vi "Add Peak and Valley Detection Settings Section.vi"(8 "error in (no error)":errorcluster, 10 "Stages":string[](array[string])=["Boost", "Battery", "Off"], 11 "Global Settings Item Ref in":T1=18446744073709551615 format="%.0x") -> (0 "error out":errorcluster, 3 "Global Settings Item Ref out":T1=18446744073709551615 format="%.0x")   [LabVIEW 2015, in "Fuel Injector Analysis Addon System Explorer.lvlib"]
uses:
  Fuel Injector Analysis Addon System Explorer.lvlib
  <vilib>/NI Veristand/Custom Device API/Custom Device Item Ref.ctl
  Shared/Types/Analysis.Channels.Select.ctl
  <vilib>/NI Veristand/Custom Device API/Custom Device Channel.ctl
  <vilib>/NI Veristand/Custom Device API/Custom Device Channel Type.ctl
  Shared/Types/Stage.PullIn.Types.ctl
  Shared/Types/Stage.Transition.Types.ctl
  Shared/Constants.vi
  <vilib>/NI Veristand/Custom Device Tools/Custom Device Utility Library/NI VeriStand - Search for Item by GUID.vi
  <vilib>/NI Veristand/Custom Device API/Custom Device API.lvlib
  Shared/Fuel Injector Analysis Addon Shared.lvlib
  <vilib>/NI Veristand/Custom Device Tools/Custom Device Utility Library/Custom Device Utility Library.lvlib
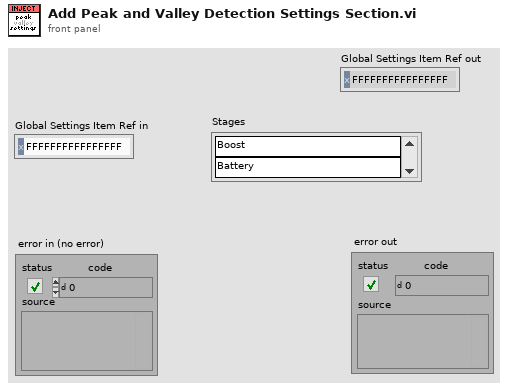
[diagram p1: front panel]
types:
  T1 = typedef "Custom Device API.lvlib/Custom Device Item Ref.ctl" = u64
  T2 = typedef "Fuel Injector Analysis Addon Shared.lvlib/Stage.Transition.Types.ctl" = enum8{"Stage Transition Inactive Time", "Stage Transition Voltage Increase", "Stage Transition Current Decrease", "Stage Transition Active Time"}
  T3 = typedef "Fuel Injector Analysis Addon Shared.lvlib/Stage.PullIn.Types.ctl" = enum8{"Pull In Transition Pulses", "Pull In Transition Current Drop"}
  T4 = typedef "Fuel Injector Analysis Addon Shared.lvlib/Analysis.Channels.Select.ctl" = cluster{"Pull In Time":bool, "Pull In Max Current":bool, "Pull In Max Voltage":bool, "Pull In Min Voltage":bool, "Pull In Avg Voltage":bool, "Hold Time":bool, "Hold Max Current":bool, "Hold Min Current":bool, "Hold Avg Current":bool, "Hold Max Voltage":bool, "Hold Min Voltage":bool, "Hold Avg Max Voltage":bool, "Hold Avg Min Voltage":bool, "Off Time":bool, "Off Max Current":bool, "Off Min Current":bool, "Off Avg Current":bool, "Off Max Voltage":bool, "Off Min Voltage":bool, "Off Avg Voltage":bool, "Total Voltage Pulses":bool, "Total Stage Time":bool}
  T5 = typedef "Custom Device API.lvlib/Custom Device Channel.ctl" = cluster{"Type":T6, "Units":string, "Default Value":dbl, "Faultable":bool, "Scalable":bool}
  T6 = typedef "Custom Device API.lvlib/Custom Device Channel Type.ctl" = enum16{"Input", "Output"}
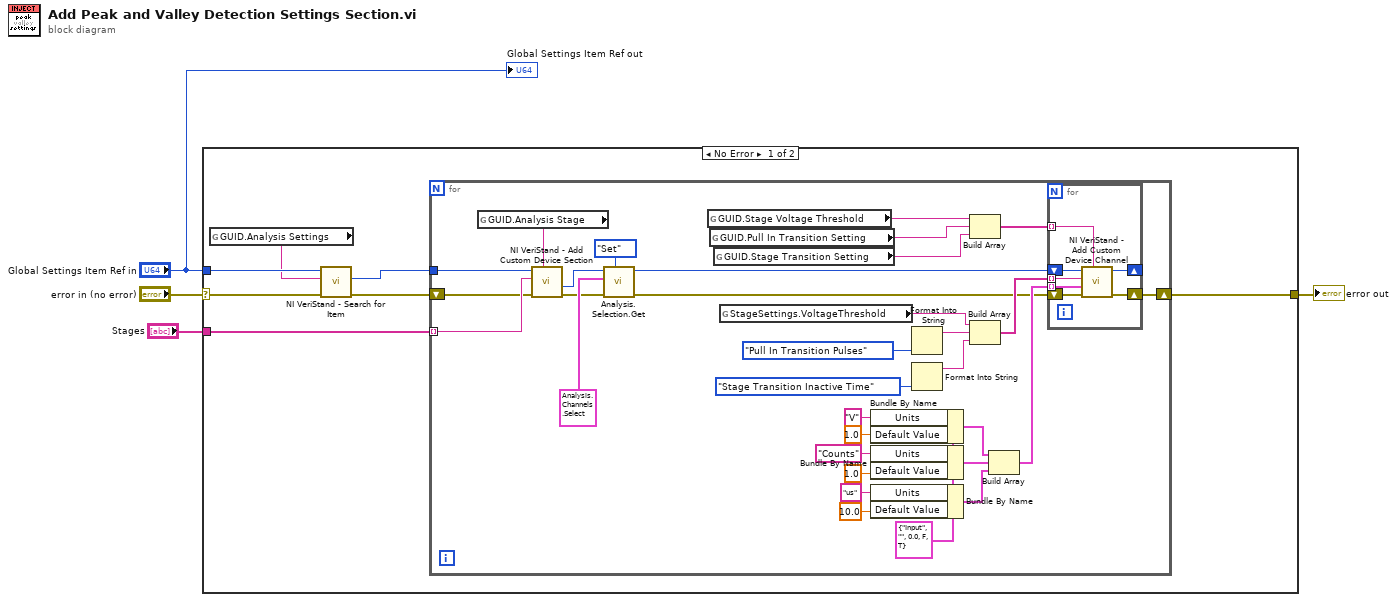
[diagram p0: block diagram]
diagram:
  n1 = case shown="No Error" "error in (no error)" {
    selector: "error in (no error)" -> [w7 w51]
    tunnel: [w11 w51] -> w3
    tunnel: "Global Settings Item Ref in" -> [w9 _]
    tunnel: "Stages" -> [w10 _]
    frame No Error {
      n2 = global read "Constants.vi" "GUID.Analysis Settings"() -> (w5:string)
      n3 = call-poly <vilib>:"NI VeriStand - Search for Item.vi"("error in"=w7, "Item GUID"=w5, "Section Ref in"=w9) -> ("error out"=w6:errorcluster, "Item Ref"=w8:T1)  [unwired: 5 in, 2 out]
      n4 = for {
        shift-right: [w31] -> w11
        shift-left: w6 -> [w41]
        tunnel: w10 -> [w42] mode=indexing
        tunnel: w8 -> [w40]
        w24 = T5 {"Type"=enum."Input", "Units"="", "Default Value"=0.0, "Faultable"=FALSE, "Scalable"=TRUE} ("Channel")
        n5 = global read "Constants.vi" "GUID.Analysis Stage"() -> (w43:string)
        n6 = call <vilib>:"NI VeriStand - Add Custom Device Section.vi"("GUID (Default Section)"=w43, "error in (no error)"=w41, "Section Name"=w42, "Parent Ref in"=w40) -> ("error out"=w37:errorcluster, "Section Ptr"=w38:T1)  [unwired: 4 in, 2 out]
        n7 = call "Analysis.Selection.Get.vi"("Action"=enum8{"Get", "Set"}."Set", "error in (no error)"=w37, "Selections"=T4 {"Pull In Time"=TRUE, "Pull In Max Current"=TRUE, "Pull In Max Voltage"=TRUE, "Pull In Min Voltage"=TRUE, "Pull In Avg Voltage"=TRUE, "Hold Time"=TRUE, "Hold Max Current"=TRUE, "Hold Min Current"=TRUE, "Hold Avg Current"=TRUE, "Hold Max Voltage"=TRUE, "Hold Min Voltage"=TRUE, "Hold Avg Max Voltage"=TRUE, "Hold Avg Min Voltage"=TRUE, "Off Time"=TRUE, "Off Max Current"=TRUE, "Off Min Current"=TRUE, "Off Avg Current"=TRUE, "Off Max Voltage"=TRUE, "Off Min Voltage"=TRUE, "Off Avg Voltage"=TRUE, "Total Voltage Pulses"=TRUE, "Total Stage Time"=TRUE} ("Analysis Options"), "Item Ref in"=w38) -> ("error out"=w18:errorcluster, "Item Ref out"=w19:T1)  [unwired: 5 in, 1 out]
        n8 = global read "Constants.vi" "GUID.Stage Voltage Threshold"() -> (w15:string)
        n9 = global read "Constants.vi" "GUID.Pull In Transition Setting"() -> (w14:string)
        n10 = global read "Constants.vi" "GUID.Stage Transition Setting"() -> (w13:string)
        n11 = global read "Constants.vi" "StageSettings.VoltageThreshold"() -> (w26:string)
        n12 = Bundle By Name(cluster=w24, "Units"="V", "Default Value"=1.0) -> (w25:T5)
        n13 = Bundle By Name(cluster=w24, "Units"="Counts", "Default Value"=1.0) -> (w32:T5)
        n14 = Bundle By Name(cluster=w24, "Units"="us", "Default Value"=10.0) -> (w33:T5)
        n15 = Format Into String(Stage.PullIn.Types."Pull In Transition Pulses" ("input 1")) -> (resulting string=w20:string)  [unwired: 3 in, 1 out]
        n16 = Format Into String(Stage.Transition.Types."Stage Transition Inactive Time" ("input 1")) -> (resulting string=w21:string)  [unwired: 3 in, 1 out]
        n17 = Build Array(w15, w14, w13) -> (w12:string[])
        n18 = Build Array(w26, w20, w21) -> (w35:string[])
        n19 = Build Array(w25, w32, w33) -> (w34:T5[])
        n20 = for {
          shift-right: [w49] -> w31
          shift-left: w18 -> [w50]
          tunnel: w34 -> [w47] mode=indexing
          tunnel: w12 -> [w46] mode=indexing
          tunnel: w35 -> [w45] mode=indexing
          shift-right: [w44] -> _
          shift-left: w19 -> [w48]
          n21 = call <vilib>:"NI VeriStand - Add Custom Device Channel.vi"("GUID (Default Channel)"=w46, "error in (no error)"=w50, "Channel"=w47, "Channel Name"=w45, "Parent Ref in"=w48) -> ("error out"=w49:errorcluster, "Parent Ref out"=w44:T1)  [unwired: 3 in, 2 out]
        }
      }
    }
    frame Error {
    }
  }
  "error out" <- w3
  "Global Settings Item Ref out" <- "Global Settings Item Ref in"
